vi "GCSArray_import.vi"(0 "GCSArray input string":string, 1 "Range":T1, 5 "error in (no error)":errorcluster) -> (14 "GCSArray data":dbl[][](array[numeric]), 19 "error out":errorcluster)   [LabVIEW 2020]
doc: "Takes an Input string, limited to a specific character Range, and tries to import as a GCSArray.\n\nFrom the GCSArray the data section is extracted using the LabVIEW regular expression engine. The numbers contained in this data block are then converted from textual representation into double values (64-bit floating point). The result of this operation is returned as a 2D double array to the caller by GCSArray data. For details of the conversion process, see the GCS Array Data Format Description (Release 1.2.1, Date: 2010-09-27, PI document code: SM146E)."
uses:
  GCSArray_regex_range.ctl
  GCSArray_regex_selector.ctl
panel:
  # "Import the textual representation of a GCSArray and\nreturn the contained numerical data as 2D double array."
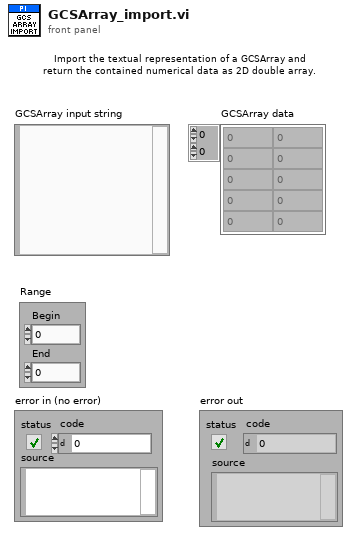
[diagram p1: front panel]
types:
  T1 = typedef "GCSArray_regex_range.ctl" = cluster{"Begin":i32, "End":i32}
  T2 = typedef "GCSArray_regex_selector.ctl" = enum16{"GCS_ARRAY Block Full", "GCS_ARRAY Block ID", "GCS_ARRAY Block Header", "GCS_ARRAY Block Data", "GCS_ARRAY Identifier", "GCS_ARRAY Remark", "GCS_ARRAY Version", "GCS_ARRAY Dimension", "GCS_ARRAY Type", "GCS_ARRAY Separator", "GCS_ARRAY NData", "GCS_ARRAY NData%", "GCS_ARRAY NData% Keyword", "GCS_ARRAY Name%", "GCS_ARRAY Name% Keyword", "GCS_ARRAY Start%", "GCS_ARRAY Start% Keyword", "GCS_ARRAY End%", "GCS_ARRAY End% Keyword", "GCS_ARRAY Delta%", "GCS_ARRAY Delta% Keword", "GCS_ARRAY Sample Time", "GCS_ARRAY Unit of transmitted value%", "GCS_ARRAY Trans_Unit% Keyword", "GCS_ARRAY Trans_Unit% = RAW Keyword", "GCS_ARRAY Unit of displayed value%", "GCS_ARRAY Disp_Unit% Keyword", "GCS_ARRAY Nominator%", "GCS_ARRAY Ratio_Nom% Keyword", "GCS_ARRAY Denominator%", "GCS_ARRAY Ratio_Denom% Keyword", "GCS_ARRAY End of Header", "GCS_ARRAY Empty line of Header"}
  T3 = typedef "GCSArray_header.ctl" = cluster{"Identifier":string, "Version":i32, "Remark":string, "Dimension":i32, "Type":enum16{"Matrix", "Table"}, "Separator":u8, "NData":i32, "NData%":i32[], "Name%":string[], "Start%":dbl[], "End%":dbl[], "Delta%":dbl[], "SampleTime":dbl, "TransmittedUnit%":string[], "DisplayedUnit%":string[], "RatioNominator%":dbl[], "RatioDenominator%":dbl[]}
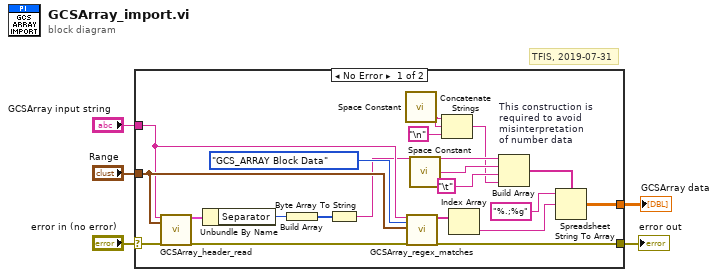
[diagram p0: block diagram]
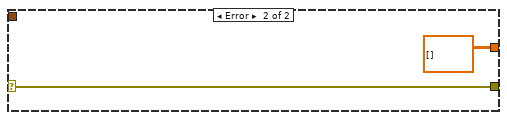
[diagram p2: hidden frame]
diagram:
  # "TFIS, 2019-07-31"
  n1 = case shown="No Error" "error in (no error)" {
    selector: "error in (no error)" -> [w21 w27]
    tunnel: [w13 w27] -> w4
    tunnel: "GCSArray input string" -> [w16 _]
    tunnel: "Range" -> [w18 _]
    tunnel: [w25 dbl[][] [] ("GCSArray data")] -> w1
    frame No Error {
      n2 = call "GCSArray_header_read.vi"("GCSArray input string"=w16, "Range"=w18, "error in (no error)"=w21) -> ("GCSArray Header"=w22:T3, "error out"=w19:errorcluster)  [unwired: 15 out]
      n3 = Unbundle By Name(w22) -> ("Separator"=w20:u8)
      n4 = Build Array(w20) -> (w23:u8[])
      n5 = Byte Array To String(unsigned byte array=w23) -> (string=w10:string)
      n6 = call "Space Constant.vi"() -> ("String"=w8:string)
      n7 = call "GCSArray_regex_matches.vi"("GCSArray input string"=w16, "Selector"=GCSArray_regex_selector."GCS_ARRAY Block Data", "Range"=w18, "error in (no error)"=w19) -> ("Matches"=w15:string[], "error out"=w13:errorcluster)  [unwired: 14 out]
      n8 = call "Space Constant.vi"() -> ("String"=w12:string)
      n9 = Concatenate Strings(w8, w8, "\n") -> (w7:string)
      n10 = Index Array(array=w15) -> (element=w14:string)  [unwired: 1 in]
      n11 = Build Array "This construction is\nrequired to avoid\nmisinterpretation\nof number data"(w10, w12, "\t", w7) -> (w11:string[])
      n12 = Spreadsheet String To Array(delimiter (Tab)=w11, format string="%.;%g", spreadsheet string=w14) -> (array=w25:dbl[][])  [unwired: 1 out]
    }
    frame Error {
    }
  }
  "error out" <- w4
  "GCSArray data" <- w1
